vi "Agilent VNA Set Sweep Time.vi"(6 "Channel":i8=1 min=1 max=99 step=1, 7 "Agilent VNA":T1, 8 "error in (no error)":errorcluster, 10 "Sweep Time, s (-1: Auto)":dbl=-1.0, 11 "VISA Resource Name":refnum<visa-resource-name>) -> (0 "error out":errorcluster, 3 "dup VISA Resource Name":refnum<visa-resource-name>)   [LabVIEW 2011]
doc: "This Vi for the HP8753B Network Analyzer is used to set averaging, smoothing, and the IF bandwidth."
uses:
  TypeDefs/Agilent VNA Instrument Info.ctl
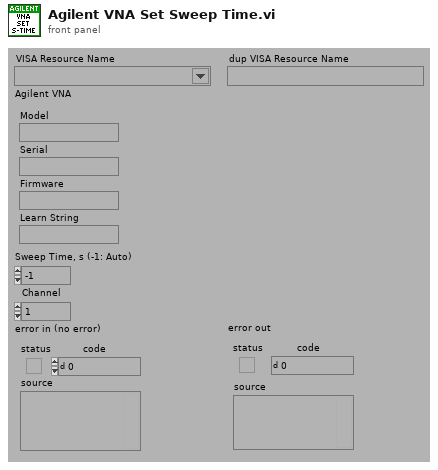
[diagram p1: front panel]
types:
  T1 = typedef "Agilent VNA Instrument Info.ctl" = cluster{"Model":string, "Serial":string, "Firmware":string, "Learn String":string}
  T2 = typedef "Agilent VNA Model.ctl" = enum16{"Not Supported", "8510X", "8719X", "8720X", "8722X", "8753X", "ENA", "PNA", "Field Fox"}
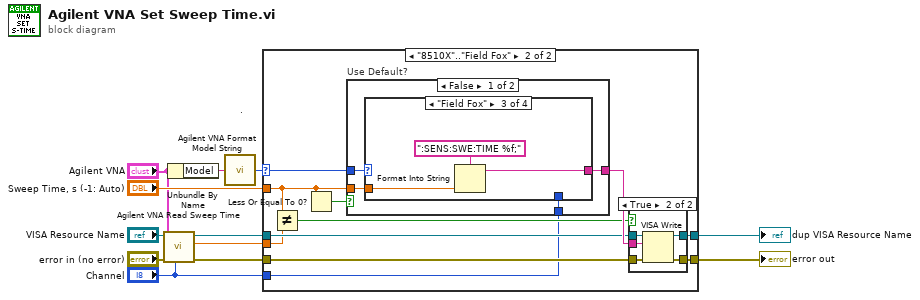
[diagram p0: block diagram]
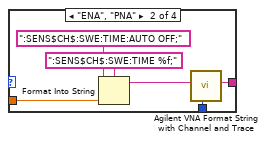
[diagram p5: hidden frame]
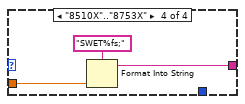
[diagram p6: hidden frame]
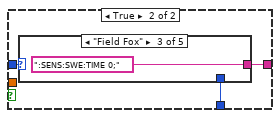
[diagram p7: hidden frame]
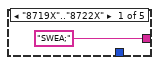
[diagram p8: hidden frame]
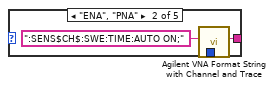
[diagram p9: hidden frame]
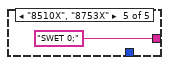
[diagram p11: hidden frame]
diagram:
  # "."
  n1 = call "Agilent VNA Read Sweep Time.vi"("Channel"="Channel", "Agilent VNA"="Agilent VNA", "error in (no error)"="error in (no error)", "VISA Resource Name"="VISA Resource Name") -> ("error out"=w7:errorcluster, "Sweep Time, s"=w6:dbl, "dup VISA Resource Name"=w8:refnum<visa-resource-name>)  [unwired: 5 out]
  n2 = Unbundle By Name("Agilent VNA") -> ("Model"=w3:string)
  n3 = call "Agilent VNA Format Model String.vi"("Model"=w3) -> ("Model"=w2:T2)
  n4 = case shown="\"8510X\"..\"Field Fox\"" w2 {
    selector: w2 -> [_ w15]
    tunnel: [w13 w25] -> w12
    tunnel: [w14 w24] -> w11
    tunnel: w8 -> [w14 w21]
    tunnel: w7 -> [w13 w20]
    tunnel: w6 -> [_ w19]
    tunnel: "Sweep Time, s (-1: Auto)" -> [_ w18]
    tunnel: "Channel" -> [_ w16]
    frame "Not Supported" {
    }
    frame "8510X".."Field Fox" {
      n5 = Not Equal?(x=w18, y=w19) -> (x != y?=w17:bool)
      n6 = Less Or Equal To 0?(x=w18) -> (x <= 0?=w23:bool)
      n7 = case "Use Default?" shown="False" w23 {
        tunnel: w18 -> [w36 _]
        tunnel: [w35 w51] -> w22
        tunnel: w15 -> [w34 w50]
        tunnel: w16 -> [w33 w49]
        frame False {
          n8 = case shown="\"Field Fox\"" w34 {
            tunnel: w36 -> [_ w41 w44 w47]
            tunnel: [_ w38 w43 w46] -> w35
            tunnel: w33 -> [_ w37 _ _]
            frame "Not Supported" {
            }
            frame "ENA", "PNA" {
              n9 = Format Into String(format string=":SENS$CH$:SWE:TIME %f;", initial string=":SENS$CH$:SWE:TIME:AUTO OFF;", w41) -> (resulting string=w39:string)  [unwired: 1 in, 1 out]
              n10 = call "Agilent VNA Format String with Channel and Trace.vi"("Channel"=w37, "String"=w39) -> ("String Out"=w38:string)  [unwired: 1 in, 6 out]
            }
            frame "Field Fox" {
              n11 = Format Into String(format string=":SENS:SWE:TIME %f;", w44) -> (resulting string=w43:string)  [unwired: 2 in, 1 out]
            }
            frame "8510X".."8753X" {
              n12 = Format Into String(format string="SWET%fs;", w47) -> (resulting string=w46:string)  [unwired: 2 in, 1 out]
            }
          }
        }
        frame True {
          n13 = case shown="\"Field Fox\"" w50 {
            tunnel: ["SWEA;" w54 ":SENS:SWE:TIME 0;" _ "SWET 0;"] -> w51
            tunnel: w49 -> [_ w53 _ _ _]
            frame "8719X".."8722X" {
            }
            frame "ENA", "PNA" {
              n14 = call "Agilent VNA Format String with Channel and Trace.vi"("Channel"=w53, "String"=":SENS$CH$:SWE:TIME:AUTO ON;") -> ("String Out"=w54:string)  [unwired: 1 in, 6 out]
            }
            frame "Field Fox" {
            }
            frame "Not Supported" {
            }
            frame "8510X", "8753X" {
            }
          }
        }
      }
      n15 = case shown="True" w17 {
        tunnel: [w26 w32] -> w25
        tunnel: [w27 w31] -> w24
        tunnel: w22 -> [_ w30]
        tunnel: w21 -> [w27 w29]
        tunnel: w20 -> [w26 w28]
        frame False {
        }
        frame True {
          n16 = VISA Write(VISA resource name=w29, write buffer=w30, error in (no error)=w28) -> (VISA resource name out=w31:refnum<visa-resource-name>, error out=w32:errorcluster)  [unwired: 1 out]
        }
      }
    }
  }
  "error out" <- w12
  "dup VISA Resource Name" <- w11
